vi "双向过零(DBL).vi"(2 "输入":dbl, 3 "复位":bool) -> (7 "双向过零":bool)   [LabVIEW 2012]
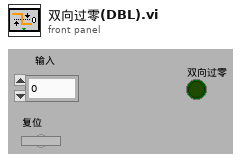
[diagram p1: front panel]
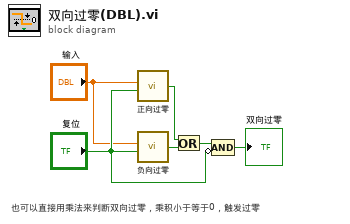
[diagram p0: block diagram]
diagram:
  # "也可以直接用乘法来判断双向过零，乘积小于等于0，触发过零"
  n1 = call-poly "正向过零.vi"("输入"="输入", "复位"="复位") -> ("正向过零"=w2:bool)  [unwired: 6 in]
  n2 = call-poly "负向过零.vi"("输入"="输入", "复位"="复位") -> ("负向过零"=w1:bool)  [unwired: 6 in]
  n3 = Or(x=w2, y=w1) -> (x .or. y?=w3:bool)
  n4 = Compound Arithmetic op=AND(w3, invert "复位") -> (→"双向过零":bool)
